vi "ITM10_Global.vi"() -> ()   [LabVIEW 2019]
panel:
  out "ITM10_Coil_B":dbl
  out "ITM10_Coil_T":dbl
  out "ITM10_Tank_B":dbl
  out "ITM10_ST":u32(colorbox)
  out "ITM10_Tank_T":dbl
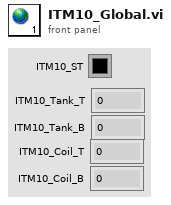
[diagram p1: front panel]
diagram:
